vi "new_analysis.vi"(10 "parameters":string[](array[string])) -> ()   [LabVIEW 2018]
doc: "SubVI that creates a new Analysis Objects and saves ID, Name, Type, Date into the private property.\nIf those data are not given a dialog appears.\nThe AnalysisObject is saved in a Queue"
uses:
  Classes/Analysis/Analysis.lvclass
  Classes/DataLoggingText/DataLogging.lvclass
  global variables.vi
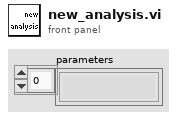
[diagram p1: front panel]
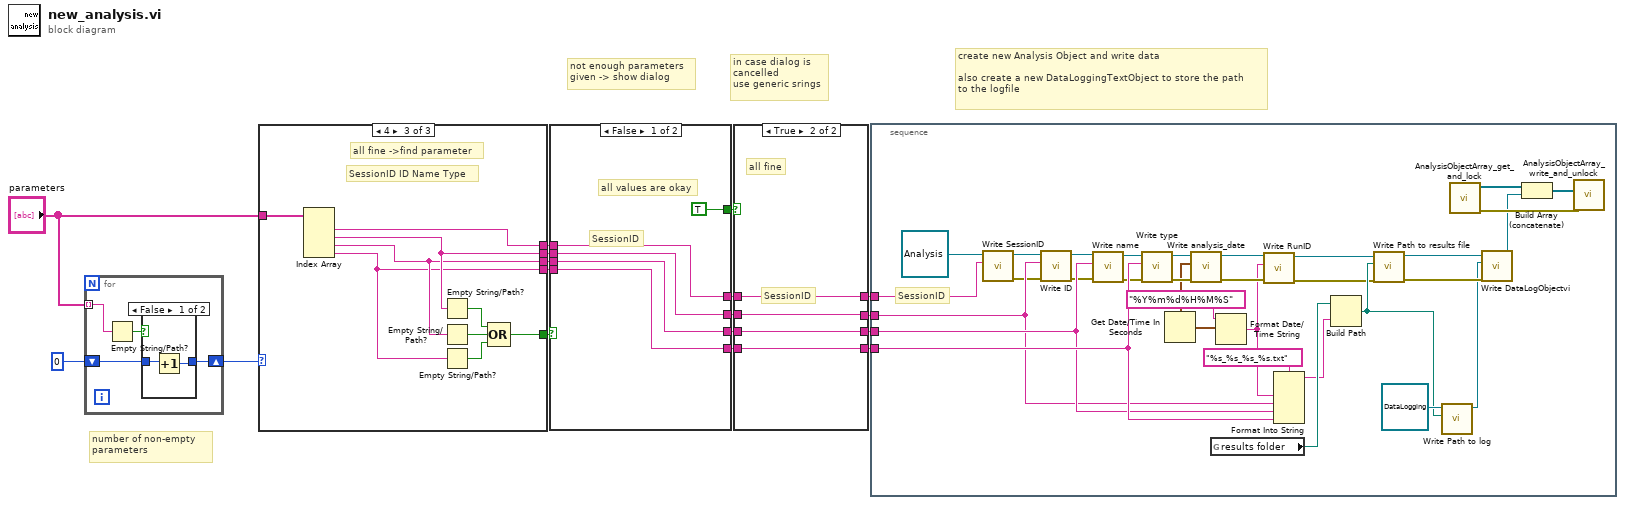
[diagram p0: block diagram]
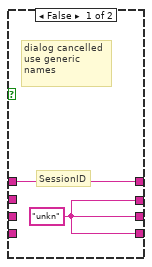
[diagram p3: hidden frame]
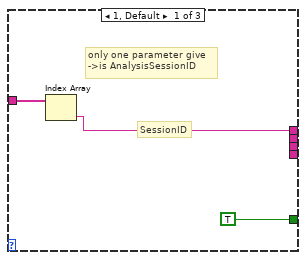
[diagram p4: hidden frame]
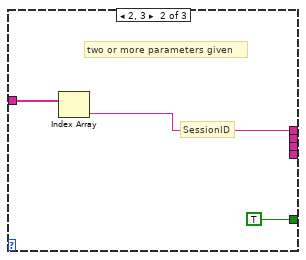
[diagram p5: hidden frame]
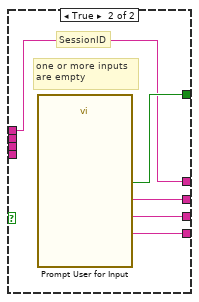
[diagram p6: hidden frame]
diagram:
  # "number of non-empty\nparameters"
  # "create new Analysis Object and write data\n\nalso create a new DataLoggingTextObject to store the path\nto the logfile"
  # "in case dialog is\ncancelled\nuse generic srings"
  # "not enough parameters\ngiven -> show dialog"
  n1 = for {
    tunnel: "parameters" -> [w21] mode=indexing
    shift-right: [w18] -> w2
    shift-left: 0 -> [w19]
    n2 = Empty String/Path?(string/path=w21) -> (empty?=w20:bool)
    n3 = case shown="False" w20 {
      tunnel: w19 -> [w22 w24]
      tunnel: [w23 w24] -> w18
      frame False {
        n4 = Increment(x=w22) -> (x+1=w23:i32)
      }
      frame True {
      }
    }
  }
  n5 = case shown="4" w2 {
    tunnel: [TRUE TRUE w36] -> w7
    tunnel: "parameters" -> [w26 w29 w35]
    tunnel: [_ _ w33] -> w8
    tunnel: [_ _ w32] -> w9
    tunnel: [_ _ w31] -> w10
    tunnel: [w25 w28 w34] -> w6
    frame 1, Default {
      # "SessionID"
      # "only one parameter give\n->is AnalysisSessionID"
      n6 = Index Array(array=w26) -> (element=w25:string)  [unwired: 1 in]
    }
    frame 2, 3 {
      # "two or more parameters given"
      # "SessionID"
      n7 = Index Array(array=w29) -> (element=w28:string)  [unwired: 1 in]
    }
    frame 4 {
      # "all fine ->find parameter"
      # "SessionID ID Name Type"
      n8 = Index Array(array=w35) -> (element #1=w34:string, element #2=w33:string, element #3=w32:string, element #4=w31:string)  [unwired: 4 in]
      n9 = Empty String/Path?(string/path=w33) -> (empty?=w38:bool)
      n10 = Empty String/Path?(string/path=w32) -> (empty?=w39:bool)
      n11 = Empty String/Path?(string/path=w31) -> (empty?=w37:bool)
      n12 = Compound Arithmetic op=OR(w38, w39, w37) -> (w36:bool)
    }
  }
  n13 = case shown="False" w7 {
    tunnel: w8 -> [w44 _]
    tunnel: w9 -> [w43 _]
    tunnel: w10 -> [w42 _]
    tunnel: [w44 w49] -> w12
    tunnel: [w43 w48] -> w13
    tunnel: [w42 w47] -> w14
    tunnel: [TRUE ("OK") w46] -> w11
    tunnel: w6 -> [w40 w45]
    tunnel: [w40 w45] -> w5
    frame False {
      # "SessionID"
      # "all values are okay"
    }
    frame True {
      # "SessionID"
      # "one or more inputs\nare empty"
      n14 = call "Prompt User for Input"() -> ("Type"=w47:string, "Name"=w48:string, "ID"=w49:string, "OK"=w46:bool)  [unwired: 15 in, 1 out]
    }
  }
  n15 = case shown="True" w11 {
    tunnel: w12 -> [_ w55]
    tunnel: w13 -> [_ w54]
    tunnel: w14 -> [_ w53]
    tunnel: [w51 w55] -> w15
    tunnel: [w51 w54] -> w16
    tunnel: [w51 w53] -> w17
    tunnel: w5 -> [w50 w52]
    tunnel: [w50 w52] -> w4
    frame False {
      w51 = "unkn"
      # "SessionID"
      # "dialog cancelled\nuse generic\nnames"
    }
    frame True {
      # "SessionID"
      # "all fine"
    }
  }
  n16 = stacked-sequence {
    tunnel: w17 -> [w85]
    tunnel: w16 -> [w84]
    tunnel: w15 -> [w83]
    tunnel: w4 -> [w62]
    frame #0 {
      # "SessionID"
      n17 = call-dynamic "Write SessionID.vi"("SessionID"=w62, "Analysis in"=refnum<class "Analysis.lvclass"> refnum ("Analysis.lvclass")) -> ("error out"=w63:errorcluster, "Analysis out"=w64:refnum<class "Analysis.lvclass">)  [unwired: 8 in]
      n18 = call-dynamic "Write ID.vi"("error in (no error)"=w63, "ID"=w83, "Analysis in"=w64) -> ("error out"=w76:errorcluster, "Analysis out"=w79:refnum<class "Analysis.lvclass">)  [unwired: 7 in]
      n19 = call-dynamic "Write name.vi"("error in (no error)"=w76, "name"=w84, "Analysis in"=w79) -> ("error out"=w75:errorcluster, "Analysis out"=w80:refnum<class "Analysis.lvclass">)  [unwired: 7 in]
      n20 = call-dynamic "Write type.vi"("error in (no error)"=w75, "type"=w85, "Analysis in"=w80) -> ("error out"=w74:errorcluster, "Analysis out"=w81:refnum<class "Analysis.lvclass">)  [unwired: 7 in]
      n21 = Get Date/Time In Seconds() -> (seconds since 1Jan1904=w66:timestamp)
      n22 = call-dynamic "Write analysis_date.vi"("error in (no error)"=w74, "analysis date"=w66, "Analysis in"=w81) -> ("error out"=w60:errorcluster, "Analysis out"=w61:refnum<class "Analysis.lvclass">)  [unwired: 7 in]
      n23 = global read "global variables.vi" "results folder"() -> (w87:path)
      n24 = Format Date/Time String(time format string (%c)="%Y%m%d%H%M%S", seconds (now)=w66) -> (date/time string=w57:string)  [unwired: 1 in]
      n25 = call-dynamic "Write RunID.vi"("error in (no error)"=w60, "RunID"=w57, "Analysis in"=w61) -> ("error out"=w58:errorcluster, "Analysis out"=w59:refnum<class "Analysis.lvclass">)  [unwired: 7 in]
      n26 = Format Into String(format string="%s_%s_%s_%s.txt", w57, w83, w84, w85) -> (resulting string=w86:string)  [unwired: 2 in, 1 out]
      n27 = Build Path(base path=w87, name or relative path=w86) -> (appended path=w68:path)
      n28 = call-dynamic "Write Path to results file.vi"("error in (no error)"=w58, "Path to results file"=w68, "Analysis in"=w59) -> ("error out"=w71:errorcluster, "Analysis out"=w72:refnum<class "Analysis.lvclass">)  [unwired: 7 in]
      n29 = call-dynamic "Write Path to log.vi"("Path to log"=w68, "DataLoggingText in"=refnum<class "DataLogging.lvclass"> refnum ("DataLoggingText.lvclass")) -> ("DataLoggingText out"=w67:refnum<class "DataLogging.lvclass">)  [unwired: 8 in, 1 out]
      n30 = call "AnalysisObjectArray_get_and_lock.vi"() -> ("error out"=w73:errorcluster, "AnalysisObjects"=w78:refnum<class "Analysis.lvclass">[])  [unwired: 10 in]
      n31 = call-dynamic "Write DataLogObjectvi.vi"("error in (no error)"=w71, "DataLogging.lvclass"=w67, "Analysis in"=w72) -> ("Analysis out"=w70:refnum<class "Analysis.lvclass">)  [unwired: 7 in, 1 out]
      n32 = Build Array (concatenate)(w78, w70) -> (w77:refnum<class "Analysis.lvclass">[])
      n33 = call "AnalysisObjectArray_write_and_unlock.vi"("error in (no error)"=w73, "AnalysisObjects"=w77) -> ()  [unwired: 9 in, 1 out]
    }
  }
